vi "Read Status Code.vi"(8 "error in (no error)":errorcluster, 11 "net-response in":refnum<class "net-response.lvclass">) -> (0 "error out":errorcluster, 2 "status code":u16, 3 "net-response out":refnum<class "net-response.lvclass">)   [LabVIEW 2020, in "net-response.lvclass"]
uses:
  net-response.lvclass
  net-response.lvclass/net-response.ctl
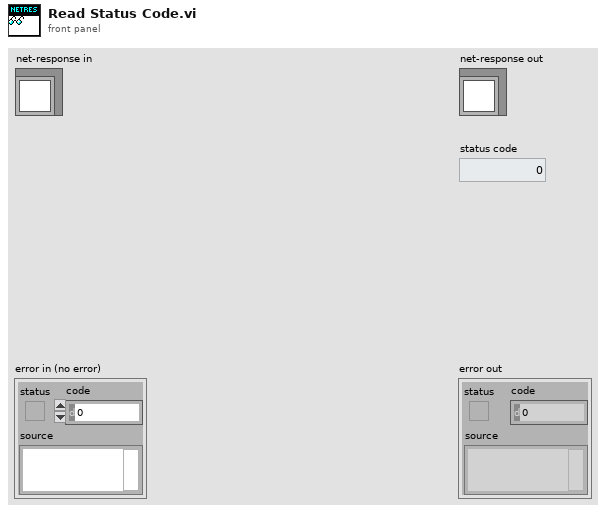
[diagram p1: front panel]
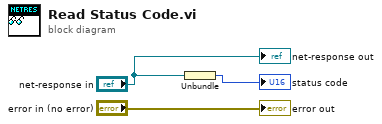
[diagram p0: block diagram]
diagram:
  n1 = Unbundle("net-response in") -> (→"status code":u16)
  "error out" <- "error in (no error)"
  "net-response out" <- "net-response in"
